vi "DEBUG Call Lib Probe.vi"() -> ()   [LabVIEW 2013]
uses:
  <vilib>/Utility/traverseref.llb/TRef TravTarget.ctl
  <vilib>/Utility/traverseref.llb/VI Scripting - Traverse.lvlib
panel:
  out "Parameter Info":T1(array[cluster])
  out "Function Name":string
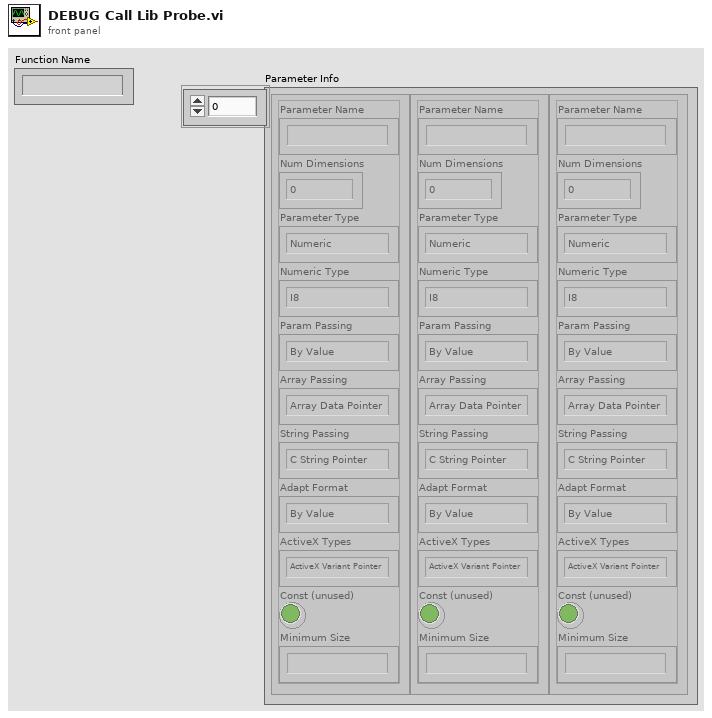
[diagram p1: front panel]
types:
  T1 = cluster{"Parameter Name":string, "Num Dimensions":i32, "Parameter Type":enum16{"Numeric", "Array", "String", "Waveform", "Digital Waveform", "Digital Table", "ActiveX", "Any", "Instance Data Pointer", "Void"}, "Numeric Type":enum16{"I8", "I16", "I32", "I64", "U8", "U16", "U32", "U64", "SGL", "DBL", "PTR INT", "PTR UINT"}, "Param Passing":enum16{"By Value", "Pointer To Value"}, "Array Passing":enum16{"Array Data Pointer", "Array Handle", "Array Handle Pointer"}, "String Passing":enum16{"C String Pointer", "Pascal String Pointer", "String Handle", "String Handle Pointer"}, "Adapt Format":enum16{"By Value", "Pointer To Value"}, "ActiveX Types":enum16{"ActiveX Variant Pointer", "IDispatch* Pointer", "IUnknown* Pointer"}, "Const (unused)":bool, "Minimum Size":string}[]
  T2 = enum32{"Invalid", "Standard", "Closed", "Hidden", "Minimized", "Maximized"}
  T3 = typedef "TRef TravTarget.ctl" = enum16{"FP", "BD", "Other"}
  T4 = enum16{"C String Pointer", "Pascal String Pointer", "String Handle", "String Handle Pointer"}
  T5 = enum16{"Numeric", "Array", "String", "Waveform", "Digital Waveform", "Digital Table", "ActiveX", "Any", "Instance Data Pointer", "Void"}
  T6 = cluster{"Parameter Name":string, "Num Dimensions":i32, "Parameter Type":enum16{"Numeric", "Array", "String", "Waveform", "Digital Waveform", "Digital Table", "ActiveX", "Any", "Instance Data Pointer", "Void"}, "Numeric Type":enum16{"I8", "I16", "I32", "I64", "U8", "U16", "U32", "U64", "SGL", "DBL", "PTR INT", "PTR UINT"}, "Param Passing":enum16{"By Value", "Pointer To Value"}, "Array Passing":enum16{"Array Data Pointer", "Array Handle", "Array Handle Pointer"}, "String Passing":enum16{"C String Pointer", "Pascal String Pointer", "String Handle", "String Handle Pointer"}, "Adapt Format":enum16{"By Value", "Pointer To Value"}, "ActiveX Types":enum16{"ActiveX Variant Pointer", "IDispatch* Pointer", "IUnknown* Pointer"}, "Const (unused)":bool, "Minimum Size":string}
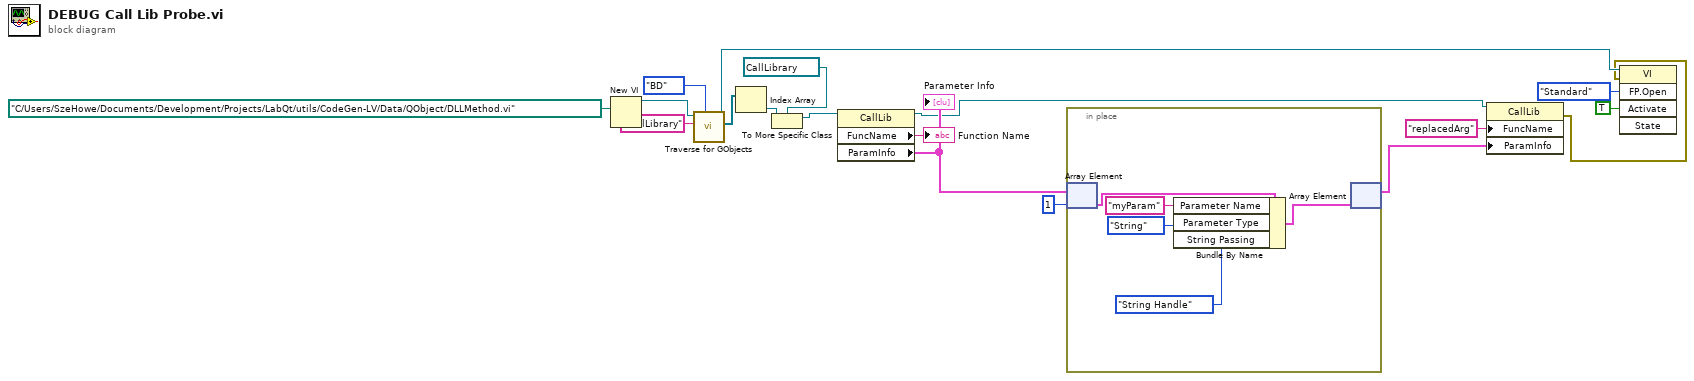
[diagram p0: block diagram]
diagram:
  n1 = New VI(10:path "C:/Users/SzeHowe/Documents/Development/Projects/LabQt/utils/CodeGen-LV/Data/QObject/DLLMethod.vi" ("template")) -> (3:w17:refnum<vi>)  [unwired: 6 in, 1 out]
  n2 = call <vilib>:"Traverse for GObjects.vi"("Traverse Target"=TRef_TravTarget."BD", "Class Name"="CallLibrary", "VI Refnum"=w17) -> ("References"=w12:refnum<vi>[], "dup VI Refnum"=w4:refnum<vi>)  [unwired: 5 in, 2 out]
  n3 = Index Array(array=w12) -> (element=w11:refnum<vi>)  [unwired: 1 in]
  n4 = To More Specific Class(target class=refnum<vi> refnum ("Replace"), reference=w11) -> (specific class reference=w14:refnum<vi>)  [unwired: 1 in, 1 out]
  n5 = property class="CallLib"(reference=w14) -> (reference out=w7:refnum<vi>, "FuncName"=→"Function Name":string, "ParamInfo"=w9:T1)  [unwired: 1 in, 1 out]
  "Parameter Info" <- w9
  n6 = in-place {
    n7 = in-place-array #1(w9, 1) -> (w23:T6)
    n8 = Bundle By Name(cluster=w23, "Parameter Name"="myParam", "Parameter Type"=T5."String", "String Passing"=T4."String Handle") -> (w19:T6)
    n9 = in-place-array #1(w19) -> (w5:T1)  [unwired: 1 out]
  }
  n10 = property class="CallLib"(reference=w7, "FuncName"="replacedArg" ("Function Name"), "ParamInfo"=w5) -> (error out=w1:errorcluster)  [unwired: 1 in, 1 out]
  n11 = invoke class="VI" method="FP.Open"(reference=w4, error in=w1, "Activate"=TRUE ("Activate?"), "State"=T2."Standard") -> ()  [unwired: 1 in, 5 out]
